vi "Store Identify Data.vi"(4 "Source (\"\")":string, 8 "error in (no error)":errorcluster, 11 "VISA resource name":refnum<visa-resource-name>) -> (0 "error out":errorcluster, 3 "VISA resource name out":refnum<visa-resource-name>)   [LabVIEW 2020, in "Yokogawa GX Series.lvlib"]
doc: "This VI logouts from the instrument. Then it can not re-login."
uses:
  <instrlib>/Yokogawa GX Series/Yokogawa GX Series.lvlib
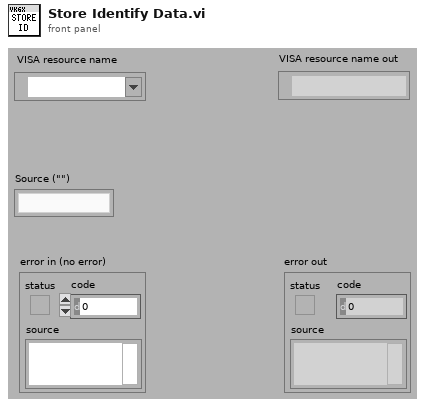
[diagram p1: front panel]
types:
  T1 = cluster{"User Name":string, "User ID":string, "Password":string, "Serial Auth Type (0: Not Auth)":u16, "SMARTDAC+ Type (0: Unknown)":u16, "Bluetooth Password":string}
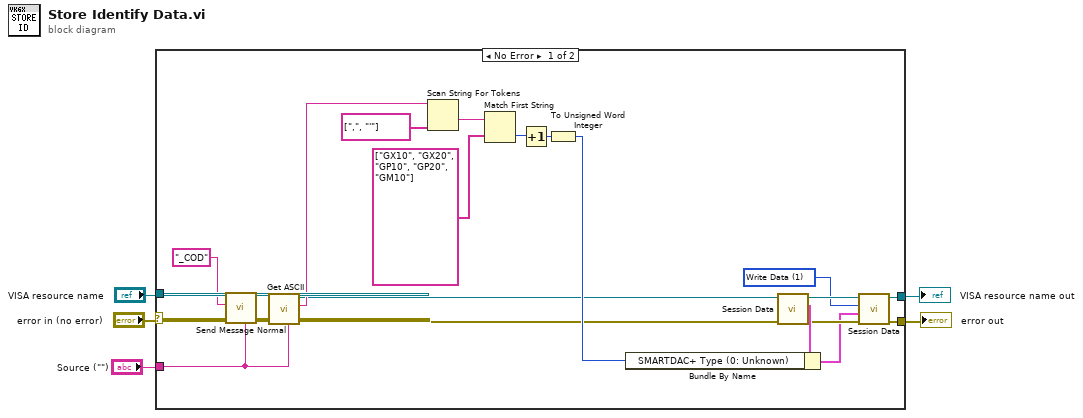
[diagram p0: block diagram]
diagram:
  n1 = case shown="No Error" "error in (no error)" {
    selector: "error in (no error)" -> [w10 w28]
    tunnel: "Source (\"\")" -> [w9 _]
    tunnel: "VISA resource name" -> [w11 w29]
    tunnel: [w22 w29] -> w2
    tunnel: [w21 w28] -> w1
    frame No Error {
      w23 = 1 items=["Read Data", "Write Data", "Clear Data", "Clear All Data"] ("Action (0 : Read Data)")
      n2 = call <instrlib>:"Send Message Normal.vi"("Source (\"\")"=w9, "error in (no error)"=w10, "Send Message (\"\")"="_COD", "VISA resource name"=w11) -> ("error out"=w18:errorcluster, "VISA resource name out"=w19:refnum<visa-resource-name>)  [unwired: 5 in, 1 out]
      n3 = call <instrlib>:"Get ASCII.vi"("Source (\"\")"=w9, "error in (no error)"=w18, "VISA resource name"=w19) -> ("error out"=w6:errorcluster, "ASCII Data"=w17:string, "VISA resource name out"=w7:refnum<visa-resource-name>)  [unwired: 6 in]
      n4 = Scan String For Tokens(6:string[] [",", "'"], 9:w17) -> (1:w15:string)  [unwired: 4 in, 3 out]
      n5 = Match First String(2:string[] ["GX10", "GX20", "GP10", "GP20", "GM10"], 3:w15) -> (0:w13:i32)  [unwired: 1 out]
      n6 = Increment(x=w13) -> (x+1=w12:i32)
      n7 = To Unsigned Word Integer(number=w12) -> (unsigned 16bit integer=w8:u16)
      n8 = call <instrlib>:"Session Data.vi"("error in (no error)"=w6, "VISA resource name"=w7) -> ("error out"=w25:errorcluster, "User Data Out"=w27:T1, "VISA resource name out"=w26:refnum<visa-resource-name>)  [unwired: 7 in]
      n9 = Bundle By Name(cluster=w27, "SMARTDAC+ Type (0: Unknown)"=w8) -> (w24:T1)
      n10 = call <instrlib>:"Session Data.vi"("error in (no error)"=w25, "User Data In"=w24, "Action (0 : Read Data)"=w23, "VISA resource name"=w26) -> ("error out"=w21:errorcluster, "VISA resource name out"=w22:refnum<visa-resource-name>)  [unwired: 5 in, 1 out]
    }
    frame Error {
    }
  }
  "error out" <- w1
  "VISA resource name out" <- w2
